vi "main.vi"() -> ()   [LabVIEW 2025]
uses:
  <vilib>/jgoebel/LabVIEW MCP Server SDK/jgoebel_lib_LabVIEW_MCP_Server_SDKMCP Server.lvlib
panel:
  out "response":string
  out "request":string
  out "Numeric":i32
  in  "stop":bool
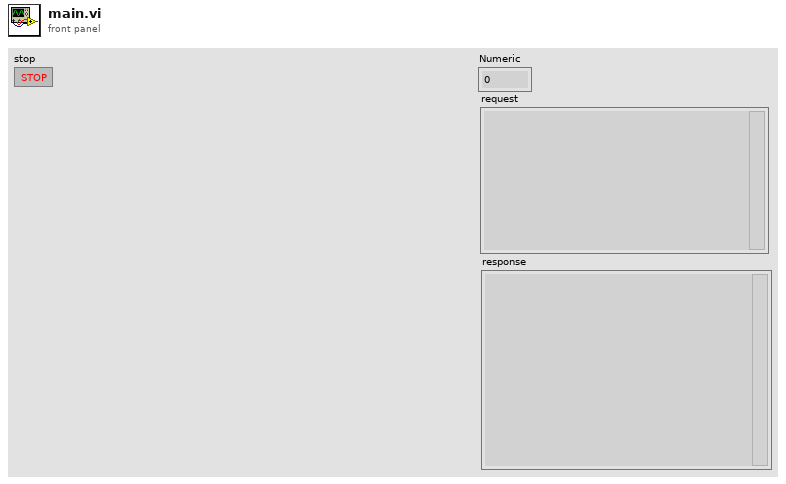
[diagram p1: front panel]
types:
  T1 = typedef "jgoebel_lib_LabVIEW_MCP_Server_SDKMCP Server.lvlib/jgoebel_lib_LabVIEW_MCP_Server_SDKUser Events.ctl" = cluster{"onError":refnum<user-event>, "onLog":refnum<user-event>, "onConnect":refnum<user-event>, "onToolsList":refnum<user-event>, "onToolsCall":refnum<user-event>, "onNotification":refnum<user-event>, "onTool":refnum<user-event>, "onRpc":refnum<user-event>}
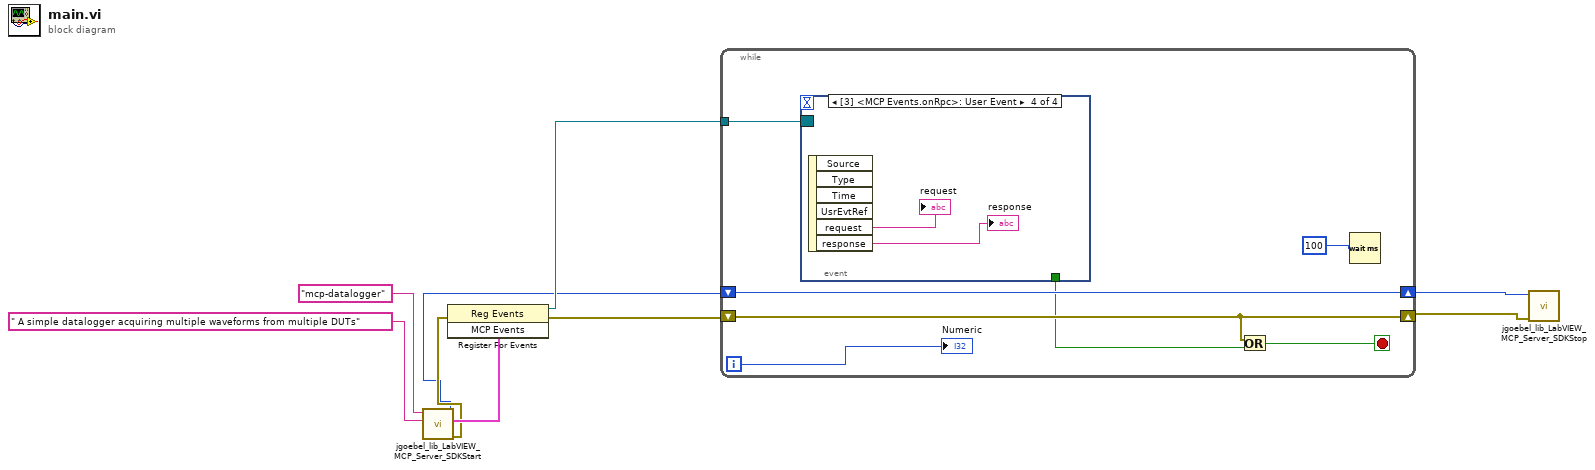
[diagram p0: block diagram]
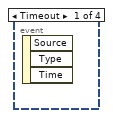
[diagram p2: hidden frame]
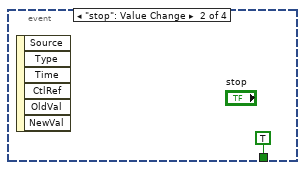
[diagram p3: hidden frame]
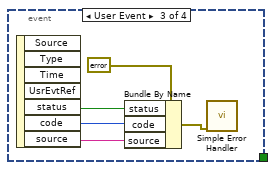
[diagram p4: hidden frame]
diagram:
  n1 = call <vilib>:"jgoebel_lib_LabVIEW_MCP_Server_SDKStart.vi"("Description"=" A simple datalogger acquiring multiple waveforms from multiple DUTs", "Name"="mcp-datalogger") -> ("error out"=w4:errorcluster, "MCP Events"=w5:T1, "id out"=w3:i32)  [unwired: 7 in]
  n2 = register-events(error in=w4, w5) -> (reference out=w8:refnum<event-registration>, error out=w9:errorcluster)  [unwired: 1 in]
  n3 = while {
    shift-right: [w16] -> w2
    shift-left: w3 -> [w16]
    shift-right: [w14] -> w1
    shift-left: w9 -> [w14]
    tunnel: w8 -> [w11]
    i -> [w13]
    stop <- w15 stop-if-true
    n4 = event shown="[3] <MCP Events.onRpc>: User Event" {
      selector: w11 -> [_ _ _ _]
      dyn-events: _ -> [_ _ _ _]
      timeout: _ -> [_ _ _ _]
      tunnel: [_ TRUE ("stop") _ _] -> w10
      event Timeout {
        n5 = event-data() -> ()  [unwired: 1 in, 3 out]
      }
      event "stop": Value Change {
        n6 = event-data() -> ()  [unwired: 1 in, 6 out]
      }
      event User Event {
        n7 = event-data() -> ("status"=w21:bool, "code"=w20:i32, "source"=w19:string)  [unwired: 1 in, 4 out]
        n8 = Bundle By Name(cluster=errorcluster {"status"=FALSE, "code"=0, "source"=""} ("error constant"), "status"=w21, "code"=w20, "source"=w19) -> (w18:errorcluster)
        n9 = call <vilib>:"Simple Error Handler.vi"("error in (no error)"=w18) -> ()  [unwired: 4 in, 5 out]
      }
      event User Event {
        n10 = event-data() -> ("request"=→"request":string, "response"=→"response":string)  [unwired: 1 in, 4 out]
      }
    }
    n11 = Or(x=w14, y=w10) -> (x .or. y?=w15:bool)
    n12 = Wait (ms)(milliseconds to wait=u32 100) -> ()  [unwired: 1 out]
    "Numeric" <- w13
  }
  n13 = call <vilib>:"jgoebel_lib_LabVIEW_MCP_Server_SDKStop.vi"("error in (no error)"=w1, "id"=w2) -> ()  [unwired: 9 in, 1 out]
